vi "Alter Table Query.vi"(8 "error in (no error)":errorcluster, 9 "Column Defintion String":string, 10 "Table Name":string, 11 "PostgreSQL in":refnum<class "PostgreSQL.lvclass">) -> (0 "error out":errorcluster, 1 "Alter Table Query":string, 3 "PostgreSQL out":refnum<class "PostgreSQL.lvclass">)   [LabVIEW 2018, in "Database.lvlib" / "PostgreSQL.lvclass"]
uses:
  PostgreSQL.lvclass
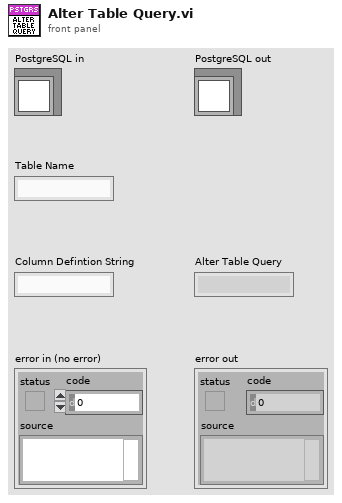
[diagram p1: front panel]
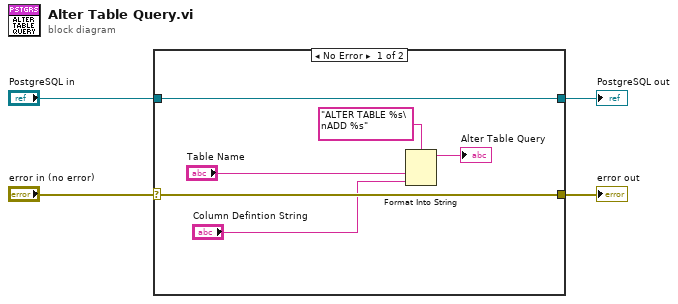
[diagram p0: block diagram]
diagram:
  n1 = case shown="No Error" "error in (no error)" {
    selector: "error in (no error)" -> [w9 w11]
    tunnel: "PostgreSQL in" -> [w10 w12]
    tunnel: [w10 w12] -> w3
    tunnel: [w9 w11] -> w1
    frame No Error {
      n2 = Format Into String(format string="ALTER TABLE %s\nADD %s", "Table Name", "Column Defintion String") -> (resulting string=→"Alter Table Query":string)  [unwired: 2 in, 1 out]
    }
    frame Error {
    }
  }
  "error out" <- w1
  "PostgreSQL out" <- w3
